vi "GetControlTerminalReference.vi"(8 "error in":errorcluster, 11 "ControlTerminal in":refnum<class "ControlTerminal.lvclass">) -> (0 "error out":errorcluster, 1 "reference":refnum<vi>, 3 "ControlTerminal out":refnum<class "ControlTerminal.lvclass">)   [LabVIEW 2014, in "Raspberry Pi Compatible Compiler for LabVIEW.lvlib" / "ControlTerminal.lvclass"]
uses:
  ControlTerminal.lvclass
  Generic/Generic.lvclass
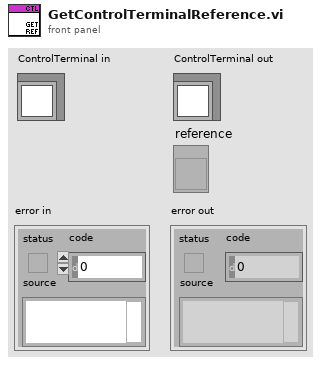
[diagram p1: front panel]
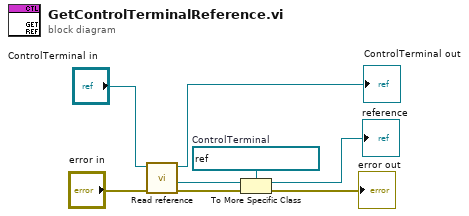
[diagram p0: block diagram]
diagram:
  w8 = refnum<vi> refnum  # ControlTerminal
  n1 = call "Read reference.vi"("error in"="error in", "GObject in"="ControlTerminal in") -> ("error out"=w6:errorcluster, "reference"=w5:refnum<vi>, "GObject out"=→"ControlTerminal out":refnum<class "ControlTerminal.lvclass">)  [unwired: 5 in]
  n2 = To More Specific Class(target class=w8, reference=w5, error in=w6) -> (specific class reference=→"reference":refnum<vi>, error out=→"error out":errorcluster)
